vi "Close Generic Object Refnum__ogtk.vi"   [LabVIEW 2016]
doc: "This VI is polymorphic to allow closing an array of refnums."
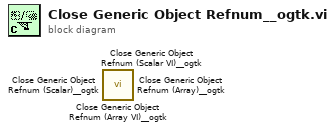
[diagram p0: block diagram]
diagram:
  n1 = call <userlib>:"Close Generic Object Refnum (Array VI)__ogtk.vi"() -> ()  [unwired: 10 in, 2 out]
  n2 = call <userlib>:"Close Generic Object Refnum (Scalar VI)__ogtk.vi"() -> ()  [unwired: 10 in, 2 out]
  n3 = call <userlib>:"Close Generic Object Refnum (Scalar)__ogtk.vi"() -> ()  [unwired: 11 in, 1 out]
  n4 = call <userlib>:"Close Generic Object Refnum (Array)__ogtk.vi"() -> ()  [unwired: 11 in, 1 out]
